vi "Example Callback - VelocityReached Callback.vi"(4 "VelocityReached":refnum<user-event>, 5 "Event Data":cluster{"sender":refnum<k24>, "velocity":i16}, 6 "Control Ref":refnum<k24>, 7 "Event Common Data":T1) -> ()   [LabVIEW 2010]
uses:
  C:/tf/play/labview/Tinkerforge.dll
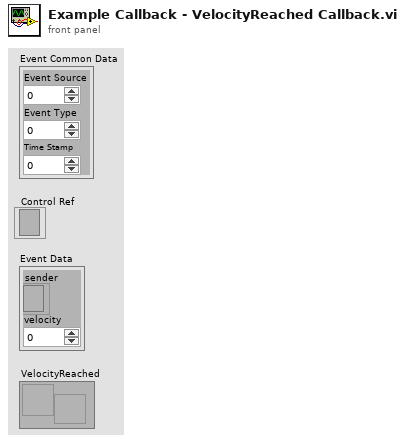
[diagram p1: front panel]
types:
  T1 = cluster{"Event Source":i32, "Event Type":u32, "Time Stamp":u32}
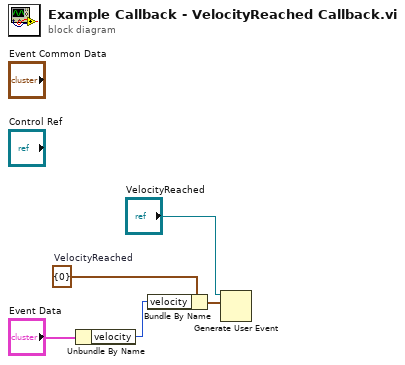
[diagram p0: block diagram]
diagram:
  w3 = cluster{"velocity":i16} {"velocity"=0}  # VelocityReached
  n1 = Unbundle By Name("Event Data") -> ("velocity"=w2:i16)
  n2 = Bundle By Name(cluster=w3, "velocity"=w2) -> (w1:cluster{"velocity":i16})
  n3 = Generate User Event(user event="VelocityReached", event data cluster=w1) -> ()  [unwired: 1 in, 2 out]
